vi "SaveOneSweep.vi"(5 "Position":T1[](array[typedef]), 7 "SectionProperties":T3, 8 "error in (no error)":errorcluster, 9 ".csv file from N5222A":string, 10 "Temperature, deg C":dbl, 11 "DataLog in":refnum<class "DataLog.lvclass">) -> (0 "error out":errorcluster, 3 "DataLog out":refnum<class "DataLog.lvclass">)   [LabVIEW 2018, in "DataLog.lvclass"]
uses:
  DataLog.lvclass
  DatalogSubvis/SearchableTag.ctl
  Sequence/SequenceSubvis/RF Direction.ctl
  Sequence/SequenceSubvis/PolarizationSelect.ctl
  APARMainSubvis/VXM Public API/singleAxisMoveDef.ctl
  APARMainSubvis/VXM Public API/mmWaveAxis.ctl
  DataLog.lvclass/DataLog.ctl
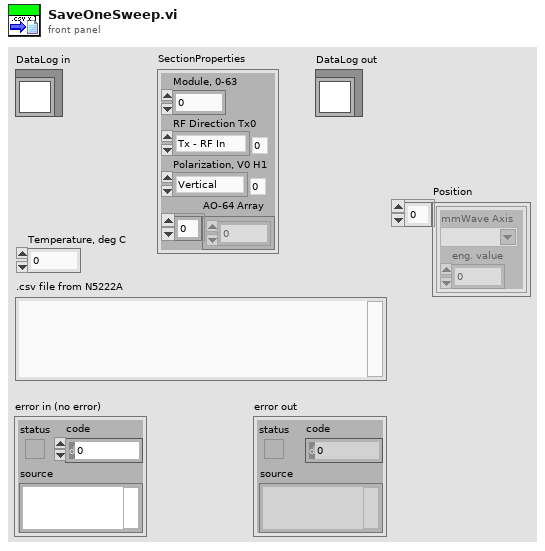
[diagram p1: front panel]
types:
  T1 = typedef "singleAxisMoveDef.ctl" = cluster{"mmWave Axis":T2, "eng. value":dbl}
  T2 = typedef "mmWaveAxis.ctl" = string
  T3 = typedef "DataLog.lvclass/SearchableTag.ctl" = cluster{"Module, 0-63":i32, "RF Direction Tx0":T4, "Polarization, V0 H1":T5, "AO-64 Array":dbl[]}
  T4 = typedef "RF Direction.ctl" = enum16{"Tx - RF In", "Rx - RF Out"}
  T5 = typedef "PolarizationSelect.ctl" = enum16{"Vertical", "Horizontal"}
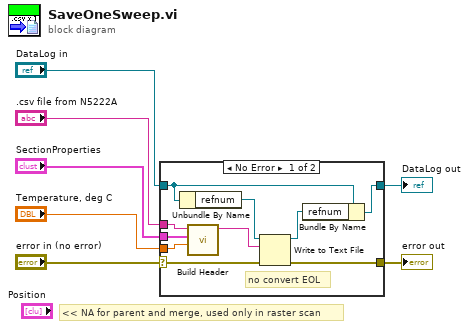
[diagram p0: block diagram]
diagram:
  # "<< NA for parent and merge, used only in raster scan"
  n1 = case shown="No Error" "error in (no error)" {
    selector: "error in (no error)" -> [w10 w19]
    tunnel: [w9 w19] -> w6
    tunnel: [w12 w18] -> w4
    tunnel: "DataLog in" -> [w13 w18]
    tunnel: ".csv file from N5222A" -> [w16 _]
    tunnel: "Temperature, deg C" -> [w15 _]
    tunnel: "SectionProperties" -> [w8 _]
    frame No Error {
      # "no convert EOL"
      n2 = Unbundle By Name(w13) -> ("refnum"=w14:refnum<file>)
      n3 = call "Build Header.vi"("Temp, deg C"=w15, "SectionProperties"=w8, "PNA .csv File"=w16) -> ("One Record"=w17:string)  [unwired: 8 in]
      n4 = Write to Text File(file (use dialog)=w14, text=w17, error in=w10) -> (refnum out=w11:refnum<file>, error out=w9:errorcluster)  [unwired: 1 in, 1 out]
      n5 = Bundle By Name(cluster=w13, "refnum"=w11) -> (w12:refnum<class "DataLog.lvclass">)
    }
    frame Error {
    }
  }
  "error out" <- w6
  "DataLog out" <- w4
